vi "UART String Test.vi"() -> ()   [LabVIEW 2017]
uses:
  <vilib>/myRIO/Instrument Drivers/Onboard IO/UART/typedef/VISA Configuration.ctl
  <vilib>/Instr/_visa.llb/VISA Configure Serial Port (Instr).vi
  <vilib>/myRIO/Instrument Drivers/Onboard IO/UART/UART.lvlib
panel:
  out "x-y":u32
  out "Array":string[](array[string])
  out "unsigned byte array":u8[](array[numeric])
  in  "input cluster":T1={"baud rate (9600)"=9600, "data bits (8)"=8, "parity (0:none)"=enum."None", "stop bits (10: 1 bit)"=10, "flow control (0:none)"=0, "termination char\n(0xA = '\\n' = LF) "=10, "Enable Termination\nChar (T)"=TRUE, "timeout (10sec)"=1000} {"termination char\n(0xA = '\\n' = LF)" format="%.0x"; "flow control (0:none)" items=["None", "XON/XOFF", "RTS/CTS", "XON/XOFF & RTS/CTS", "DTR/DSR", "XON/XOFF & DTR/DSR"]; "stop bits (10: 1 bit)" items=["1.0"=10, "1.5"=15, "2.0"=20]; "data bits (8)" min=5 max=8 step=1}
  in  "stop":bool
  out "error out":errorcluster
  in  "error in (no error)":errorcluster
  out "Characters Read":string
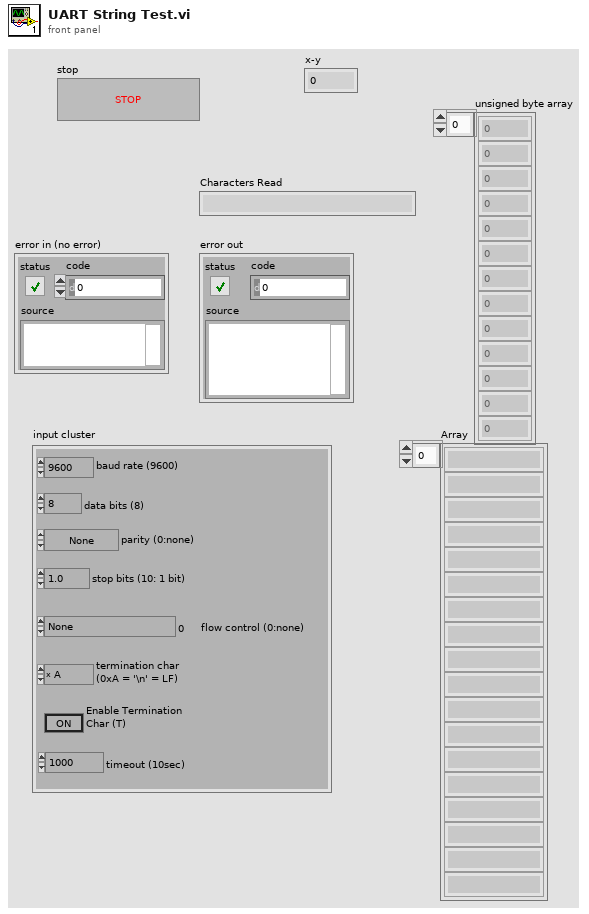
[diagram p1: front panel]
types:
  T1 = typedef "UART.lvlib/VISA Configuration.ctl" = cluster{"baud rate (9600)":u32, "data bits (8)":u16, "parity (0:none)":enum16{"None", "Odd", "Even", "Mark", "Space"}, "stop bits (10: 1 bit)":u16, "flow control (0:none)":u16, "termination char\n(0xA = '\\n' = LF) ":u8, "Enable Termination\nChar (T)":bool, "timeout (10sec)":u32}
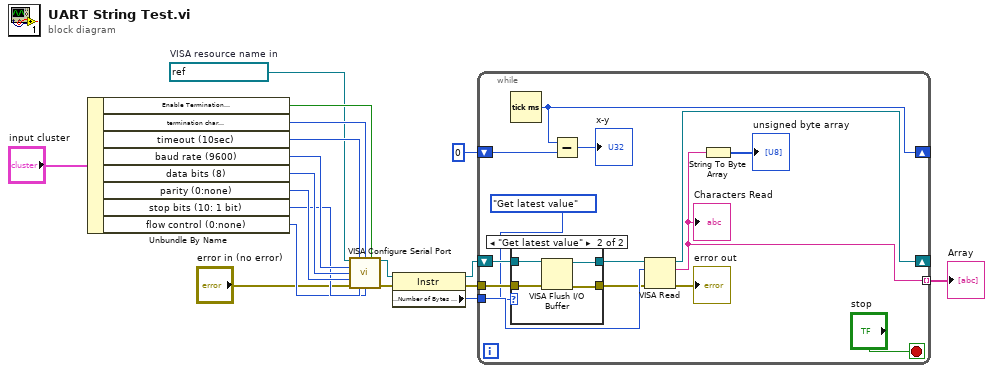
[diagram p0: block diagram]
diagram:
  w9 = refnum<visa-resource-name> "ASRL2::INSTR"  # VISA resource name in
  n1 = Unbundle By Name("input cluster") -> ("Enable Termination\nChar (T)"=w11:bool, "termination char\n(0xA = '\\n' = LF)"=w12:u8, "timeout (10sec)"=w13:u32, "baud rate (9600)"=w18:u32, "data bits (8)"=w17:u16, "parity (0:none)"=w16:enum16{"None", "Odd", "Even", "Mark", "Space"}, "stop bits (10: 1 bit)"=w15:u16, "flow control (0:none)"=w14:u16)
  n2 = call-poly "VISA Configure Serial Port"("VISA resource name"=w9, "timeout (10sec)"=w13, "termination char\n(0xA = '\\n' = LF)"=w12, "Enable Termination\nChar (T)"=w11, "baud rate (9600)"=w18, "data bits (8)"=w17, "parity (0:none)"=w16, "error in (no error)"="error in (no error)", "stop bits (10: 1 bit)"=w15, "flow control (0:none)"=w14) -> ("VISA resource name out"=w4:refnum<visa-resource-name>, "error out"=w6:errorcluster)  [unwired: 4 in]
  n3 = property class="Instr"(reference=w4, error in=w6) -> (reference out=w3:refnum<visa-resource-name>, error out=w5:errorcluster, "Serial Settings:Number of Bytes at Serial Port"=w2:u32)
  n4 = while {
    tunnel: w5 -> [w26]
    tunnel: [w29] -> w7 mode=indexing
    tunnel: w2 -> [w28]
    shift-right: [w23] -> _
    shift-left: w3 -> [w27]
    shift-right: [w20] -> _
    shift-left: u32 0 -> [w21]
    stop <- "stop" stop-if-true
    n5 = Tick Count (ms)() -> (millisecond timer value=w20:u32)
    n6 = case shown="\"Get latest value\"" enum16{"Read all", "Get latest value"}."Get latest value" {
      tunnel: w27 -> [w34 w38]
      tunnel: w26 -> [w33 w37]
      tunnel: [w33 w35] -> w25
      tunnel: [w34 w36] -> w24
      frame "Read all", Default {
      }
      frame "Get latest value" {
        n7 = VISA Flush I/O Buffer(VISA resource name=w38, error in (no error)=w37) -> (VISA resource name out=w36:refnum<visa-resource-name>, error out=w35:errorcluster)  [unwired: 1 in]
      }
    }
    n8 = Subtract(x=w20, y=w21) -> (x-y=→"x-y":u32)
    n9 = VISA Read(VISA resource name=w24, byte count=w28, error in (no error)=w25) -> (VISA resource name out=w23:refnum<visa-resource-name>, read buffer=w29:string, error out=→"error out":errorcluster)  [unwired: 1 out]
    "Characters Read" <- w29
    n10 = String To Byte Array(string=w29) -> (unsigned byte array=→"unsigned byte array":u8[])
  }
  "Array" <- w7
